vi "Start Arduino Comms.vi"(1 "Resource index":i32) -> (0 "Error":errorcluster)   [LabVIEW 2018]
uses:
  <vilib>/Instr/_visa.llb/VISA Open Access Mode.ctl
  Arduino_comms_Global.vi
  <vilib>/Instr/_visa.llb/VISA Configure Serial Port (Instr).vi
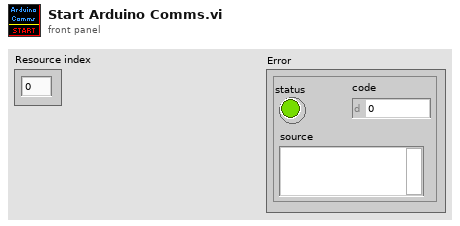
[diagram p1: front panel]
types:
  T1 = typedef "Arduino Config & resource typedef.ctl" = cluster{"baud rate (bps)":u32, "timeout (ms)":u32, "data bits":u16, "parity":enum16{"None", "Odd", "Even", "Mark", "Space"}, "stop bits (10: 1 bit)":u16, "flow control":u16, "termination char (hex)":u8, "Enable Termination Char":bool, "byte count":u32, "Resource locked?":bool}
  T2 = typedef "VISA Open Access Mode.ctl" = u32
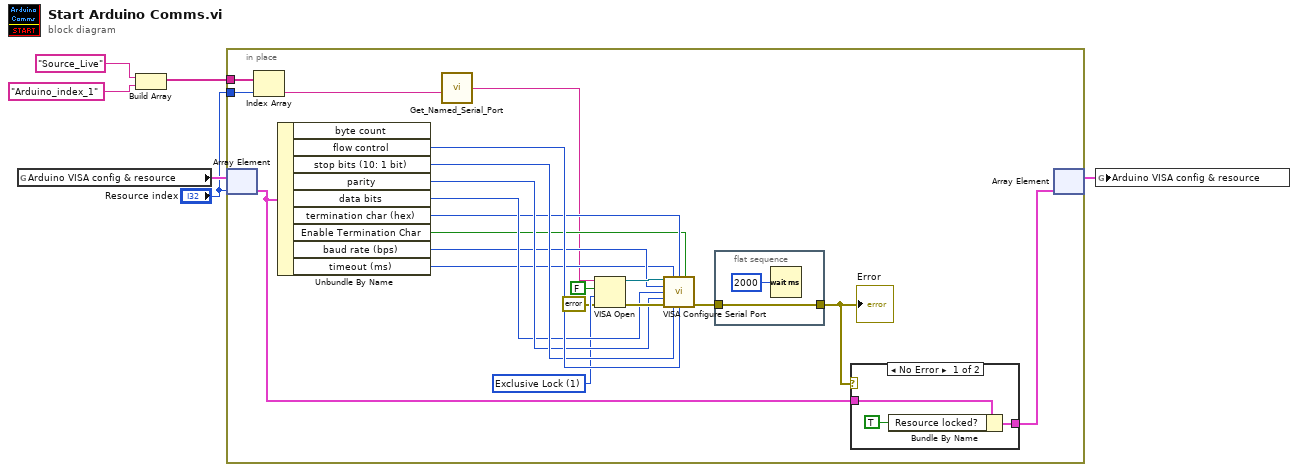
[diagram p0: block diagram]
diagram:
  n1 = global read "Arduino_comms_Global.vi" "Arduino VISA config & resource"() -> (w6:T1[])
  n2 = Build Array("Source_Live" ("Serial Port Alias"), "Arduino_index_1" ("Serial Port Alias")) -> (w2:string[])
  n3 = in-place {
    in-place-border: w2 -> [w10]
    in-place-border: "Resource index" -> [w9]
    w17 = T2 1 items=["VISA Defaults"=0, "Exclusive Lock"=1, "Load Configured Settings"=4] ("Access Mode")
    n4 = in-place-array #1(w6, "Resource index") -> (w12:T1)
    n5 = Index Array(array=w10, index=w9) -> (element=w8:string)
    n6 = Unbundle By Name(w12) -> ("flow control"=w25:u16, "stop bits (10: 1 bit)"=w24:u16, "parity"=w23:enum16{"None", "Odd", "Even", "Mark", "Space"}, "data bits"=w22:u16, "termination char (hex)"=w19:u8, "Enable Termination Char"=w18:bool, "baud rate (bps)"=w21:u32, "timeout (ms)"=w20:u32)  [unwired: 1 out]
    n7 = call "Get_Named_Serial_Port.vi"("Serial Port Alias"=w8) -> ("Serial Port Name"=w7:string)
    n8 = VISA Open(duplicate session (F)=FALSE, access mode=w17, error in (no error)=errorcluster {"status"=FALSE, "code"=0, "source"=""}, VISA resource name=w7) -> (VISA resource name=w27:refnum<visa-resource-name>, error out=w26:errorcluster)  [unwired: 1 in]
    n9 = call-poly "VISA Configure Serial Port"("VISA resource name"=w27, "timeout (10sec)"=w20, "termination char\n(0xA = '\\n' = LF)"=w19, "Enable Termination\nChar (T)"=w18, "baud rate (9600)"=w21, "data bits (8)"=w22, "parity (0:none)"=w23, "error in (no error)"=w26, "stop bits (10: 1 bit)"=w24, "flow control (0:none)"=w25) -> ("error out"=w14:errorcluster)  [unwired: 4 in, 1 out]
    n10 = flat-sequence {
      tunnel: w14 -> [w28]
      tunnel: [w28] -> w13
      frame #0 {
        n11 = Wait (ms)(milliseconds to wait=u32 2000) -> ()  [unwired: 1 out]
      }
    }
    n12 = case shown="No Error" w13 {
      tunnel: [w30 w33] -> w11
      tunnel: w12 -> [w31 w33]
      frame No Error {
        n13 = Bundle By Name(cluster=w31, "Resource locked?"=TRUE ("Locked")) -> (w30:T1)
      }
      frame Error {
      }
    }
    n14 = in-place-array #1(w11) -> (w5:T1[])  [unwired: 1 out]
    "Error" <- w13
  }
  n15 = global write "Arduino_comms_Global.vi" "Arduino VISA config & resource"(w5) -> ()
